vi "New File Logger.vi"(6 "Level":T6, 7 "Logger Name":string, 8 "error in (no error)":errorcluster, 9 "General Options":T2, 10 "Filetype":string, 11 "File Options":T1) -> (0 "error out":errorcluster)   [LabVIEW 2016, in "Global_logger.lvlib"]
uses:
  Global_logger.lvlib
  Levels.ctl
  General Options.ctl
  Log Fields.ctl
  Level Meaning.ctl
  Sorting.ctl
  File Options.ctl
  Logger Output.ctl
  Logger Type.ctl
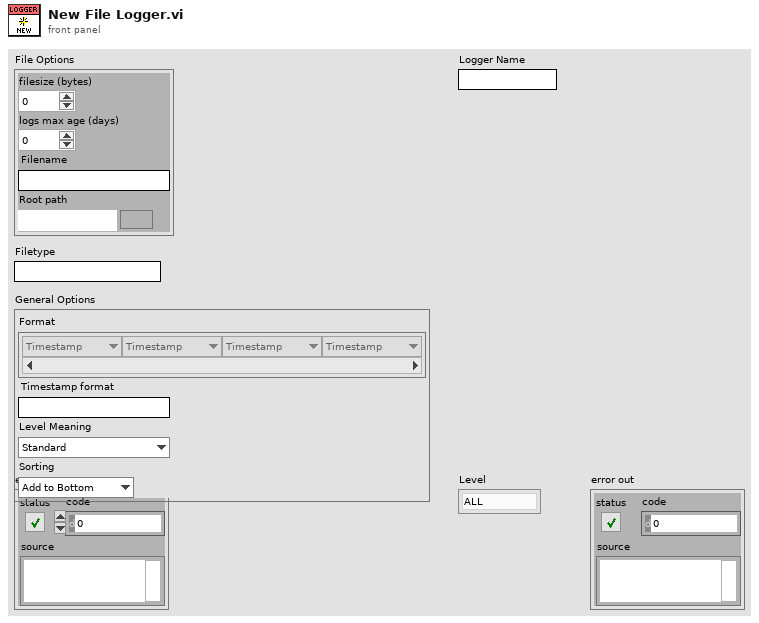
[diagram p1: front panel]
types:
  T1 = typedef "Global_logger.lvlib/File Options.ctl" = cluster{"filesize (bytes)":u32, "logs max age (days) ":i32, "Filename":string, "Root path":path}
  T2 = typedef "Global_logger.lvlib/General Options.ctl" = cluster{"Format":T3[], "Timestamp format":string, "Level Meaning":T4, "Sorting":T5}
  T3 = typedef "Global_logger.lvlib/Log Fields.ctl" = enum16{"Timestamp", "Level", "Message", "Source VI", "Source App", "Logger Name"}
  T4 = typedef "Global_logger.lvlib/Level Meaning.ctl" = enum16{"Standard", "Positive", "Exact"}
  T5 = typedef "Global_logger.lvlib/Sorting.ctl" = enum16{"Add to Bottom", "Add to Top"}
  T6 = typedef "Global_logger.lvlib/Levels.ctl" = enum16{"ALL", "TRACE", "DEBUG", "INFO", "WARN", "ERROR", "FATAL", "OFF"}
  T7 = typedef "Global_logger.lvlib/Logger Type.ctl" = enum16{"FILE", "UI"}
  T8 = typedef "Global_logger.lvlib/Logger Output.ctl" = cluster{"Level":T6, "Level Meaning":T4, "Sorting":T5, "Type":T7, "Filetype":string, "Filename":string, "Root path":path, "Max filesize (bytes)":i32, "Max age (days)":i32, "Ctl Refnum":refnum<vi>, "String Ctl Delimiter":string, "Format":T3[], "Timestamp format":string}
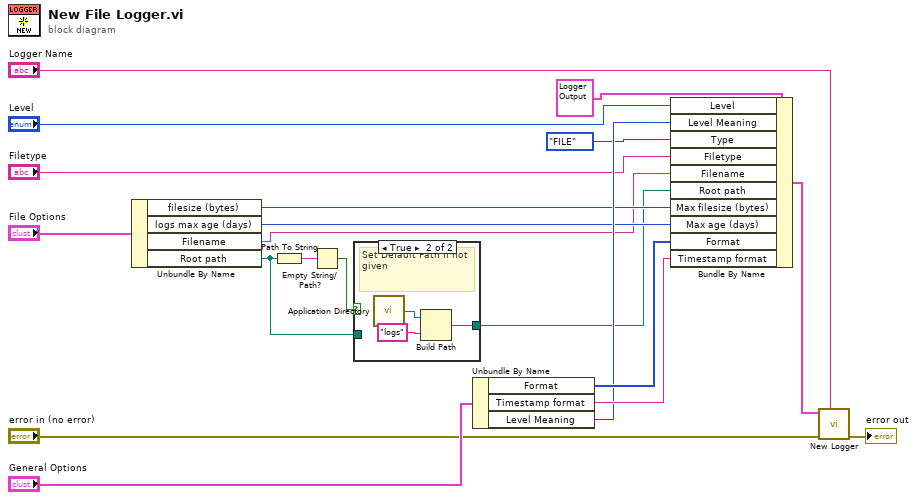
[diagram p0: block diagram]
diagram:
  n1 = Unbundle By Name("File Options") -> ("filesize (bytes)"=w8:u32, "logs max age (days)"=w7:i32, "Filename"=w6:string, "Root path"=w2:path)
  n2 = Path To String(path=w2) -> (string=w4:string)
  n3 = Empty String/Path?(string/path=w4) -> (empty?=w1:bool)
  n4 = case shown="True" w1 {
    tunnel: [w21 w22] -> w3
    tunnel: w2 -> [w21 _]
    frame False {
    }
    frame True {
      # "Set Default Path If not given"
      n5 = call <vilib>:"Application Directory.vi"() -> ("Application Directory"=w24:path)
      n6 = Build Path(base path=w24, name or relative path="logs") -> (appended path=w22:path)
    }
  }
  n7 = Unbundle By Name("General Options") -> ("Format"=w16:T3[], "Timestamp format"=w15:string, "Level Meaning"=w14:T4)
  n8 = Bundle By Name(cluster=T8 {"Level"=enum."ALL", "Level Meaning"=enum."Standard", "Sorting"=enum."Add to Bottom", "Type"=enum."FILE", "Filetype"="", "Filename"="", "Root path"=path "", "Max filesize (bytes)"=0, "Max age (days)"=0, "Ctl Refnum"=refnum, "String Ctl Delimiter"="", "Format"=[], "Timestamp format"=""} ("Logger Output"), "Level"="Level", "Level Meaning"=w14, "Type"=Logger_Type."FILE", "Filetype"="Filetype", "Filename"=w6, "Root path"=w3, "Max filesize (bytes)"=w8, "Max age (days)"=w7, "Format"=w16, "Timestamp format"=w15) -> (w18:T8)
  n9 = call "New Logger.vi"("Logger Name"="Logger Name", "error in (no error)"="error in (no error)", "Logger Output in"=w18) -> ("error out"=→"error out":errorcluster)  [unwired: 8 in]
